vi "PythonName.vi"(6 "add self":bool=TRUE, 8 "error in":errorcluster, 11 "Constant in":refnum<class "Constant.lvclass">) -> (0 "error out":errorcluster, 3 "Constant out":refnum<class "Constant.lvclass">, 5 "name":string, 7 "UID":string)   [LabVIEW 2014, in "Constant.lvclass"]
uses:
  Constant.lvclass
  Python/Parsing/Python Functions.lvlib
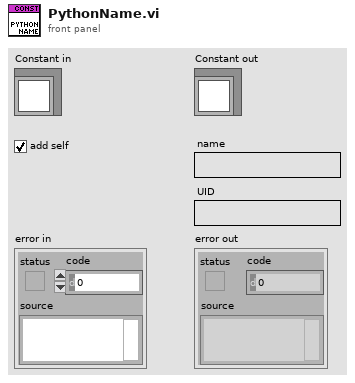
[diagram p1: front panel]
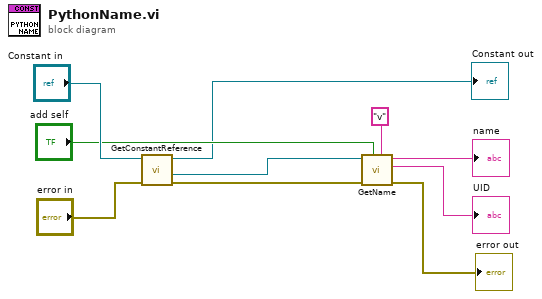
[diagram p0: block diagram]
diagram:
  n1 = call "GetConstantReference.vi"("error in"="error in", "Constant in"="Constant in") -> ("error out"=w4:errorcluster, "reference out"=w8:refnum<vi>, "Constant out"=→"Constant out":refnum<class "Constant.lvclass">)  [unwired: 5 in]
  n2 = call "GetName.vi"("base name"="v", "add self"="add self", "error in"=w4, "GObj Refnum"=w8) -> ("error out"=→"error out":errorcluster, "UID"=→"UID":string, "name"=→"name":string)  [unwired: 5 in]
